vi "Eat.vi"(8 "error in (no error)":errorcluster caption="错误输入（无错误）", 10 "字符串":string, 11 "sheep 输入":refnum<class "sheep.lvclass">) -> (0 "error out":errorcluster caption="错误输出", 2 "字符串 2":string, 3 "sheep 输出":refnum<class "sheep.lvclass">)   [LabVIEW 2020, in "sheep.lvclass"]
uses:
  sheep.lvclass
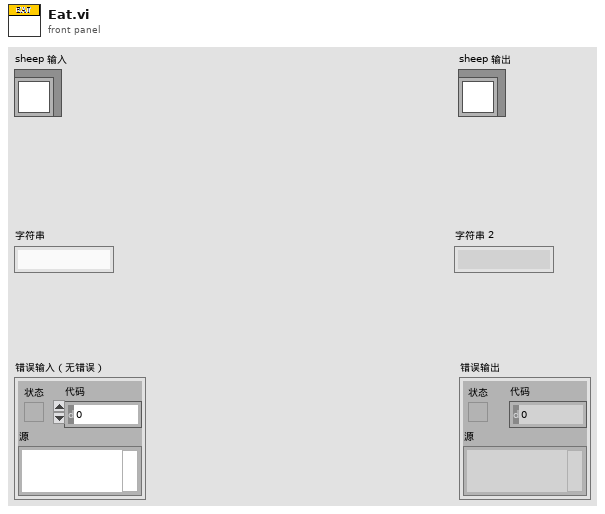
[diagram p1: front panel]
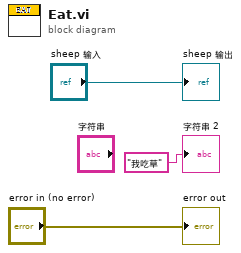
[diagram p0: block diagram]
diagram:
  "error out" <- "error in (no error)"
  "sheep 输出" <- "sheep 输入"
  "字符串 2" <- "我吃草" ("字符串 2")
